vi "WILT Agilent Correct Same Voltages.vi"(11 "Standard Agilent Data":dbl[](array[numeric])=[0.0150789, 0.0067017, 0.0050262, 0.0050262, 0.0016755, 0.0067017, 0.0050262, -0.003351, -0.0050262, 0.0050262, 0.0067017, -0.0016755, 0.0134034, 0.0016755, 0.0100527, 0.0150789, 0.003351, 0.0016755, 0.0083772, 0.0150789, 0.0050262, 0.0083772, 0.0083772, 0.0100527, 0.0150789, 0.0067017, 0.0016755, 0.003351, 0.0016755, 0.0016755, 0.0134034, 0.0016755, -0.0217806, -0.0284823, 0.003351, -0.0050262, -0.0067017, 0.0134034, 0.0083772, 0.0016755, -0.0016755, 0.003351, 0.105552, 0.0234561, 0.0134034, 0.0150789, -0.0016755, -0.0016755, 0.003303, 0.0066063, -0.0016515, -0.0066063, 0.0148638, 0.0099093, -0.0016515, 0.0148638, 0.0066063, 0.003303, -0.0379854, -0.0016515, -0.0082578, -0.0049545, -0.003303, 0.0016515, -0.809256, 238.79767, 259.98711, 242.03472, 0.776226, 135.72431, 1.271691, 169.51505, 130.6045, 132.20651, 236.32036, 235.99005, 234.30546, 236.88188, -264.32902, -207.73094, 1220.801, 77.65, 348.401, 79.079, 79.717, 80.026, 78.786, 79.191, 78.937, 79.038, 80.017, 80.836, 79.409, 78.471, 79.011, 79.04, 80.102, 77.803, 77.346, 79.36, 76.685, 77.029, 77.321, 77.89, 77.27, 76.943, 78.032, 77.108, 77.549, 77.348, 79.619, 78.244, 241.03483, 243.97762, 240.40768, -3.071427, 0.0149331, 0.0099555, 0.0066369, 0.0049776, -0.0033186, 0.0, 0.0099555, 0.0082962, 0.0116148, 0.0049776, 0.0, 0.0165924, 0.0116148, 0.0033186, 0.0033186, -0.0049776, 0.0066369, 0.0066369, 0.0049776, 0.0099555, 0.0033186, 0.0165924, 0.0066369, 0.0232296, 0.0, 0.0945771, 0.0929178, 0.0016593, 0.0, 0.0099555, 0.0033186, 0.0082962, 0.0033186, 0.0099555, 0.0099555, 0.0082962, -0.0066369, -0.0116148, 0.0016593, 0.0049776, 0.0033186, 0.0066369, 0.0099555, 0.0116148, 0.0, 0.0149331, 0.0016593, 0.0066369, 77.454, 77.456, 77.632, 77.638, 77.159, 75.814, 77.922, 78.196, 78.44, 79.124, 79.366, 79.841, 80.354, 80.293, 80.037, 80.15, 79.992, 80.199, 79.751, 79.949, 80.23, 80.523, 80.593, 1072.373, 237.01965, 236.79856, 236.81435, 238.04611, 230.03965, 0.536922, 9.9e+37, 235.66154, 9.9e+37, 199.4982, 9.9e+37, 236.13531, 3.742653, 0.410586, -2.526687, -0.900132, 236.76698, 199.4982]) -> (3 "Corrected Agilent Data":dbl[](array[numeric])=[0.0150789, 0.0067017, 0.0050262, 0.0050262, 0.0016755, 0.0067017, 0.0050262, -0.003351, -0.0050262, 0.0050262, 0.0067017, -0.0016755, 0.0134034, 0.0016755, 0.0100527, 0.0150789, 0.003351, 0.0016755, 0.0083772, 0.0150789, 0.0050262, 0.0083772, 0.0083772, 0.0100527, 0.0150789, 0.0067017, 0.0016755, 0.003351, 0.0016755, 0.0016755, 0.0134034, 0.0016755, -0.0217806, -0.0284823, 0.003351, -0.0050262, -0.0067017, 0.0134034, 0.0083772, 0.0016755, -0.0016755, 0.003351, 0.105552, 0.0234561, 0.0134034, 0.0150789, -0.0016755, -0.0016755, 0.003303, 0.0066063, -0.0016515, -0.0066063, 0.0148638, 0.0099093, -0.0016515, 0.0148638, 0.0066063, 0.003303, -0.0379854, -0.0016515, -0.0082578, -0.0049545, -0.003303, 0.0016515, -0.809256, 238.79767, 259.98711, 242.03472, 0.776226, 135.72431, 1.271691, 169.51505, 130.6045, 132.20651, 236.32036, 236.32036, 236.32036, 235.99005, 235.99005, 235.99005, 234.30546, 234.30546, 234.30546, 236.88188, 236.88188, 236.88188, -264.32902, -207.73094, 1220.801, 77.65, 348.401, 79.079, 79.717, 80.026, 78.786, 79.191, 78.937, 79.038, 80.017, 80.836, 79.409, 78.471, 79.011, 79.04, 80.102, 77.803, 77.346, 79.36, 76.685, 77.029, 77.321, 77.89, 77.27, 76.943, 78.032, 77.108, 77.549, 77.348, 79.619, 78.244, 241.03483, 243.97762, 240.40768, -3.071427, 0.0149331, 0.0099555, 0.0066369, 0.0049776, -0.0033186, 0.0, 0.0099555, 0.0082962, 0.0116148, 0.0049776, 0.0, 0.0165924, 0.0116148, 0.0033186, 0.0033186, -0.0049776, 0.0066369, 0.0066369, 0.0049776, 0.0099555, 0.0033186, 0.0165924, 0.0066369, 0.0232296, 0.0, 0.0945771, 0.0929178, 0.0016593, 0.0, 0.0099555, 0.0033186, 0.0082962, 0.0033186, 0.0099555, 0.0099555, 0.0082962, -0.0066369, -0.0116148, 0.0016593, 0.0049776, 0.0033186, 0.0066369, 0.0099555, 0.0116148, 0.0, 0.0149331, 0.0016593, 0.0066369, 77.454, 77.456, 77.632, 77.638, 77.159, 75.814, 77.922, 78.196, 78.44, 79.124, 79.366, 79.841, 80.354, 80.293, 80.037, 80.15, 79.992, 80.199, 79.751, 79.949, 80.23, 80.523, 80.593, 1072.373, 237.01965, 237.01965, 237.01965, 236.79856, 236.79856, 236.79856, 236.81435, 236.81435, 236.81435, 238.04611, 238.04611, 238.04611, 230.03965, 230.03965, 230.03965, 0.536922, 9.9e+37, 235.66154, 235.66154, 235.66154, 9.9e+37, 199.4982, 9.9e+37, 236.13531, 236.13531, 236.13531, 3.742653, 0.410586, -2.526687, -0.900132, 236.76698, 236.76698, 236.76698, 199.4982])   [LabVIEW 2016]
uses:
  <vilib>/Utility/file.llb/Read From Spreadsheet File (string).vi
panel:
  out "Array":string[][](array[string])=[["LV Index", "Agilent", "Channel", "Station", "Sensor", "LV Data"], ["64", "2", "201", "5", "Volts", "-0.809256"], ["65", "2", "202", "6", "Volts", "238.797670"], ["66", "2", "203", "7", "Volts", "259.987110"], ["67", "2", "204", "8", "Volts", "242.034720"], ["68", "2", "205", "9", "Volts", "0.776226"], ["69", "2", "206", "10", "Volts", "135.724310"], ["70", "2", "207", "11", "Volts", "1.271691"], ["71", "2", "208", "12", "Volts", "169.515050"], ["72", "2", "209", "13", "Volts", "130.604500"], ["73", "2", "210", "14", "Volts", "132.206510"], ["74", "2", "211", "21", "Volts", "236.320360"], ["75", "2", "212", "24", "Volts", "235.990050"], ["76", "2", "213", "27", "Volts", "234.305460"], ["77", "2", "214", "30", "Volts", "236.881880"], ["78", "2", "215", "15", "Volts", "-264.329020"], ["79", "2", "216", "16", "Volts", "-207.730940"], ["112", "3", "313", "1", "Volts", "241.034830"], ["113", "3", "314", "2", "Volts", "243.977620"], ["114", "3", "315", "3", "Volts", "240.407680"], ["115", "3", "316", "4", "Volts", "-3.071427"], ["188", "6", "205", "33", "Volts", "237.019650"], ["189", "6", "206", "36", "Volts", "236.798560"], ["190", "6", "207", "39", "Volts", "236.814350"], ["191", "6", "208", "42", "Volts", "238.046110"], ["192", "6", "209", "45", "Volts", "230.039650"], ["193", "6", "210", "45", "Volts (208)", "0.536922"], ["195", "6", "212", "48", "Volts", "235.661540"], ["197", "6", "214", "51", "Volts (208)", "199.498200"], ["199", "6", "216", "54", "Volts", "236.135310"], ["200", "6", "301", "17", "Volts", "3.742653"], ["201", "6", "302", "18", "Volts", "0.410586"], ["202", "6", "303", "19", "Volts", "-2.526687"], ["203", "6", "304", "20", "Volts", "-0.900132"], ["204", "6", "305", "51", "Volts", "236.766980"], ["205", "6", "306", "48", "Volts (208)", "199.498200"]]
  in  "Initial Output Array 2":string[][](array[string])=[["LV Index", "Agilent", "Channel", "Station", "Sensor", "LV Data"], ["0", "1", "101", "1", "L1 Current", "0.015079"], ["1", "1", "102", "1", "L2 Current", "0.006702"], ["2", "1", "103", "2", "L1 Current", "0.005026"], ["3", "1", "104", "2", "L2 Current", "0.005026"], ["4", "1", "105", "3", "L1 Current", "0.001675"], ["5", "1", "106", "3", "L2 Current", "0.006702"], ["6", "1", "107", "4", "L1 Current", "0.005026"], ["7", "1", "108", "4", "L2 Current", "-0.003351"], ["8", "1", "109", "5", "L1 Current", "-0.005026"], ["9", "1", "110", "5", "L2 Current", "0.005026"], ["10", "1", "111", "6", "L1 Current", "0.006702"], ["11", "1", "112", "6", "L2 Current", "-0.001675"], ["12", "1", "113", "7", "L1 Current", "0.013403"], ["13", "1", "114", "7", "L2 Current", "0.001675"], ["14", "1", "115", "8", "L1 Current", "0.010053"], ["15", "1", "116", "8", "L2 Current", "0.015079"], ["16", "1", "201", "9", "L1 Current", "0.003351"], ["17", "1", "202", "9", "L2 Current", "0.001675"], ["18", "1", "203", "10", "L1 Current", "0.008377"], ["19", "1", "204", "10", "L2 Current", "0.015079"], ["20", "1", "205", "11", "L1 Current", "0.005026"], ["21", "1", "206", "11", "L2 Current", "0.008377"], ["22", "1", "207", "12", "L1 Current", "0.008377"], ["23", "1", "208", "12", "L2 Current", "0.010053"], ["24", "1", "209", "13", "L1 Current", "0.015079"], ["25", "1", "210", "13", "L2 Current", "0.006702"], ["26", "1", "211", "14", "L1 Current", "0.001675"], ["27", "1", "212", "14", "L2 Current", "0.003351"], ["28", "1", "213", "15", "L1 Current", "0.001675"], ["29", "1", "214", "15", "L2 Current", "0.001675"], ["30", "1", "215", "16", "L1 Current", "0.013403"], ["31", "1", "216", "16", "L2 Current", "0.001675"], ["32", "1", "301", "17", "L1 Current", "-0.021781"], ["33", "1", "302", "17", "L2 Current", "-0.028482"], ["34", "1", "303", "18", "L1 Current", "0.003351"], ["35", "1", "304", "18", "L2 Current", "-0.005026"], ["36", "1", "305", "19", "L1 Current", "-0.006702"], ["37", "1", "306", "19", "L2 Current", "0.013403"], ["38", "1", "307", "20", "L1 Current", "0.008377"], ["39", "1", "308", "20", "L2 Current", "0.001675"], ["40", "1", "309", "21", "L1 Current", "-0.001675"], ["41", "1", "310", "21", "L2 Current", "0.003351"], ["42", "1", "311", "22", "L1 Current", "0.105552"], ["43", "1", "312", "22", "L2 Current", "0.023456"], ["44", "1", "313", "23", "L1 Current", "0.013403"], ["45", "1", "314", "23", "L2 Current", "0.015079"], ["46", "1", "315", "24", "L1 Current", "-0.001675"], ["47", "1", "316", "24", "L2 Current", "-0.001675"], ["48", "2", "101", "25", "L1 Current", "0.003303"], ["49", "2", "102", "25", "L2 Current", "0.006606"], ["50", "2", "103", "26", "L1 Current", "-0.001651"], ["51", "2", "104", "26", "L2 Current", "-0.006606"], ["52", "2", "105", "27", "L1 Current", "0.014864"], ["53", "2", "106", "27", "L2 Current", "0.009909"], ["54", "2", "107", "28", "L1 Current", "-0.001651"], ["55", "2", "108", "28", "L2 Current", "0.014864"], ["56", "2", "109", "29", "L1 Current", "0.006606"], ["57", "2", "110", "29", "L2 Current", "0.003303"], ["58", "2", "111", "30", "L1 Current", "-0.037985"], ["59", "2", "112", "30", "L2 Current", "-0.001651"], ["60", "2", "113", "31", "L1 Current", "-0.008258"], ["61", "2", "114", "31", "L2 Current", "-0.004954"], ["62", "2", "115", "32", "L1 Current", "-0.003303"], ["63", "2", "116", "32", "L2 Current", "0.001651"], ["64", "2", "201", "5", "Volts", "-0.809256"], ["65", "2", "202", "6", "Volts", "238.797670"], ["66", "2", "203", "7", "Volts", "259.987110"], ["67", "2", "204", "8", "Volts", "242.034720"], ["68", "2", "205", "9", "Volts", "0.776226"], ["69", "2", "206", "10", "Volts", "135.724310"], ["70", "2", "207", "11", "Volts", "1.271691"], ["71", "2", "208", "12", "Volts", "169.515050"], ["72", "2", "209", "13", "Volts", "130.604500"], ["73", "2", "210", "14", "Volts", "132.206510"], ["74", "2", "211", "21", "Volts", "236.320360"], ["75", "2", "212", "24", "Volts", "235.990050"], ["76", "2", "213", "27", "Volts", "234.305460"], ["77", "2", "214", "30", "Volts", "236.881880"], ["78", "2", "215", "15", "Volts", "-264.329020"], ["79", "2", "216", "16", "Volts", "-207.730940"], ["80", "3", "201", "1", "Temperature", "1220.801000"], ["81", "3", "202", "2", "Temperature", "77.650000"], ["82", "3", "203", "3", "Temperature", "348.401000"], ["83", "3", "204", "4", "Temperature", "79.079000"], ["84", "3", "205", "5", "Temperature", "79.717000"], ["85", "3", "206", "6", "Temperature", "80.026000"], ["86", "3", "207", "7", "Temperature", "78.786000"], ["87", "3", "208", "8", "Temperature", "79.191000"], ["88", "3", "209", "9", "Temperature", "78.937000"], ["89", "3", "210", "10", "Temperature", "79.038000"], ["90", "3", "211", "11", "Temperature", "80.017000"], ["91", "3", "212", "12", "Temperature", "80.836000"], ["92", "3", "213", "13", "Temperature", "79.409000"], ["93", "3", "214", "14", "Temperature", "78.471000"], ["94", "3", "215", "15", "Temperature", "79.011000"], ["95", "3", "216", "16", "Temperature", "79.040000"], ["96", "3", "217", "17", "Temperature", "80.102000"], ["97", "3", "218", "18", "Temperature", "77.803000"], ["98", "3", "219", "19", "Temperature", "77.346000"], ["99", "3", "220", "20", "Temperature", "79.360000"], ["100", "3", "301", "21", "Temperature", "76.685000"], ["101", "3", "302", "22", "Temperature", "77.029000"], ["102", "3", "303", "23", "Temperature", "77.321000"], ["103", "3", "304", "24", "Temperature", "77.890000"], ["104", "3", "305", "25", "Temperature", "77.270000"], ["105", "3", "306", "26", "Temperature", "76.943000"], ["106", "3", "307", "27", "Temperature", "78.032000"], ["107", "3", "308", "28", "Temperature", "77.108000"], ["108", "3", "309", "29", "Temperature", "77.549000"], ["109", "3", "310", "30", "Temperature", "77.348000"], ["110", "3", "311", "31", "Temperature", "79.619000"], ["111", "3", "312", "32", "Temperature", "78.244000"], ["112", "3", "313", "1", "Volts", "241.034830"], ["113", "3", "314", "2", "Volts", "243.977620"], ["114", "3", "315", "3", "Volts", "240.407680"], ["115", "3", "316", "4", "Volts", "-3.071427"], ["116", "4", "101", "33", "L1 Current", "0.014933"], ["117", "4", "102", "33", "L2 Current", "0.009956"], ["118", "4", "103", "34", "L1 Current", "0.006637"], ["119", "4", "104", "34", "L2 Current", "0.004978"], ["120", "4", "105", "35", "L1 Current", "-0.003319"], ["121", "4", "106", "35", "L2 Current", "0.000000"], ["122", "4", "107", "36", "L1 Current", "0.009956"], ["123", "4", "108", "36", "L2 Current", "0.008296"], ["124", "4", "109", "37", "L1 Current", "0.011615"], ["125", "4", "110", "37", "L2 Current", "0.004978"], ["126", "4", "111", "38", "L1 Current", "0.000000"], ["127", "4", "112", "38", "L2 Current", "0.016592"], ["128", "4", "113", "39", "L1 Current", "0.011615"], ["129", "4", "114", "39", "L2 Current", "0.003319"], ["130", "4", "115", "40", "L1 Current", "0.003319"], ["131", "4", "116", "40", "L2 Current", "-0.004978"], ["132", "4", "201", "41", "L1 Current", "0.006637"], ["133", "4", "202", "41", "L2 Current", "0.006637"], ["134", "4", "203", "42", "L1 Current", "0.004978"], ["135", "4", "204", "42", "L2 Current", "0.009956"], ["136", "4", "205", "43", "L1 Current", "0.003319"], ["137", "4", "206", "43", "L2 Current", "0.016592"], ["138", "4", "207", "44", "L1 Current", "0.006637"], ["139", "4", "208", "44", "L2 Current", "0.023230"], ["140", "4", "209", "45", "L1 Current", "0.000000"], ["141", "4", "210", "45", "L2 Current", "0.094577"], ["142", "4", "211", "46", "L1 Current", "0.092918"], ["143", "4", "212", "46", "L2 Current", "0.001659"], ["144", "4", "213", "47", "L1 Current", "0.000000"], ["145", "4", "214", "47", "L2 Current", "0.009956"], ["146", "4", "215", "48", "L1 Current", "0.003319"], ["147", "4", "216", "48", "L2 Current", "0.008296"], ["148", "4", "301", "49", "L1 Current", "0.003319"], ["149", "4", "302", "49", "L2 Current", "0.009956"], ["150", "4", "303", "50", "L1 Current", "0.009956"], ["151", "4", "304", "50", "L2 Current", "0.008296"], ["152", "4", "305", "51", "L1 Current", "-0.006637"], ["153", "4", "306", "51", "L2 Current", "-0.011615"], ["154", "4", "307", "52", "L1 Current", "0.001659"], ["155", "4", "308", "52", "L2 Current", "0.004978"], ["156", "4", "309", "53", "L1 Current", "0.003319"], ["157", "4", "310", "53", "L2 Current", "0.006637"], ["158", "4", "311", "54", "L1 Current", "0.009956"], ["159", "4", "312", "54", "L2 Current", "0.011615"], ["160", "4", "313", "55", "L1 Current", "0.000000"], ["161", "4", "314", "55", "L2 Current", "0.014933"], ["162", "4", "315", "56", "L1 Current", "0.001659"], ["163", "4", "316", "56", "L2 Current", "0.006637"], ["164", "6", "101", "33", "Temperature", "77.454000"], ["165", "6", "102", "34", "Temperature", "77.456000"], ["166", "6", "103", "35", "Temperature", "77.632000"], ["167", "6", "104", "36", "Temperature", "77.638000"], ["168", "6", "105", "37", "Temperature", "77.159000"], ["169", "6", "106", "38", "Temperature", "75.814000"], ["170", "6", "107", "39", "Temperature", "77.922000"], ["171", "6", "108", "40", "Temperature", "78.196000"], ["172", "6", "109", "41", "Temperature", "78.440000"], ["173", "6", "110", "42", "Temperature", "79.124000"], ["174", "6", "111", "43", "Temperature", "79.366000"], ["175", "6", "112", "44", "Temperature", "79.841000"], ["176", "6", "113", "45", "Temperature", "80.354000"], ["177", "6", "114", "46", "Temperature", "80.293000"], ["178", "6", "115", "47", "Temperature", "80.037000"], ["179", "6", "116", "48", "Temperature", "80.150000"], ["180", "6", "117", "49", "Temperature", "79.992000"], ["181", "6", "118", "50", "Temperature", "80.199000"], ["182", "6", "119", "51", "Temperature", "79.751000"], ["183", "6", "120", "52", "Temperature", "79.949000"], ["184", "6", "201", "53", "Temperature", "80.230000"], ["185", "6", "202", "54", "Temperature", "80.523000"], ["186", "6", "203", "55", "Temperature", "80.593000"], ["187", "6", "204", "56", "Temperature", "1072.373000"], ["188", "6", "205", "33", "Volts", "237.019650"], ["189", "6", "206", "36", "Volts", "236.798560"], ["190", "6", "207", "39", "Volts", "236.814350"], ["191", "6", "208", "42", "Volts", "238.046110"], ["192", "6", "209", "45", "Volts", "230.039650"], ["193", "6", "210", "45", "Volts (208)", "0.536922"], ["194", "6", "211", "45", "SW (208)", "98999999999999993400000000000000000000.000000"], ["195", "6", "212", "48", "Volts", "235.661540"], ["196", "6", "213", "48", "SW (208)", "98999999999999993400000000000000000000.000000"], ["197", "6", "214", "51", "Volts (208)", "199.498200"], ["198", "6", "215", "51", "SW (208)", "98999999999999993400000000000000000000.000000"], ["199", "6", "216", "54", "Volts", "236.135310"], ["200", "6", "301", "17", "Volts", "3.742653"], ["201", "6", "302", "18", "Volts", "0.410586"], ["202", "6", "303", "19", "Volts", "-2.526687"], ["203", "6", "304", "20", "Volts", "-0.900132"], ["204", "6", "305", "51", "Volts", "236.766980"], ["205", "6", "306", "48", "Volts (208)", "199.498200"]]
  out "Final output array":string[][](array[string])=[["LabView Array Index", "Agilent", "Channel", "Station", "Sensor", "LV Data"], ["0", "1", "101", "1", "L1 Current", "0.015079"], ["1", "1", "102", "1", "L2 Current", "0.006702"], ["2", "1", "103", "2", "L1 Current", "0.005026"], ["3", "1", "104", "2", "L2 Current", "0.005026"], ["4", "1", "105", "3", "L1 Current", "0.001675"], ["5", "1", "106", "3", "L2 Current", "0.006702"], ["6", "1", "107", "4", "L1 Current", "0.005026"], ["7", "1", "108", "4", "L2 Current", "-0.003351"], ["8", "1", "109", "5", "L1 Current", "-0.005026"], ["9", "1", "110", "5", "L2 Current", "0.005026"], ["10", "1", "111", "6", "L1 Current", "0.006702"], ["11", "1", "112", "6", "L2 Current", "-0.001675"], ["12", "1", "113", "7", "L1 Current", "0.013403"], ["13", "1", "114", "7", "L2 Current", "0.001675"], ["14", "1", "115", "8", "L1 Current", "0.010053"], ["15", "1", "116", "8", "L2 Current", "0.015079"], ["16", "1", "201", "9", "L1 Current", "0.003351"], ["17", "1", "202", "9", "L2 Current", "0.001675"], ["18", "1", "203", "10", "L1 Current", "0.008377"], ["19", "1", "204", "10", "L2 Current", "0.015079"], ["20", "1", "205", "11", "L1 Current", "0.005026"], ["21", "1", "206", "11", "L2 Current", "0.008377"], ["22", "1", "207", "12", "L1 Current", "0.008377"], ["23", "1", "208", "12", "L2 Current", "0.010053"], ["24", "1", "209", "13", "L1 Current", "0.015079"], ["25", "1", "210", "13", "L2 Current", "0.006702"], ["26", "1", "211", "14", "L1 Current", "0.001675"], ["27", "1", "212", "14", "L2 Current", "0.003351"], ["28", "1", "213", "15", "L1 Current", "0.001675"], ["29", "1", "214", "15", "L2 Current", "0.001675"], ["30", "1", "215", "16", "L1 Current", "0.013403"], ["31", "1", "216", "16", "L2 Current", "0.001675"], ["32", "1", "301", "17", "L1 Current", "-0.021781"], ["33", "1", "302", "17", "L2 Current", "-0.028482"], ["34", "1", "303", "18", "L1 Current", "0.003351"], ["35", "1", "304", "18", "L2 Current", "-0.005026"], ["36", "1", "305", "19", "L1 Current", "-0.006702"], ["37", "1", "306", "19", "L2 Current", "0.013403"], ["38", "1", "307", "20", "L1 Current", "0.008377"], ["39", "1", "308", "20", "L2 Current", "0.001675"], ["40", "1", "309", "21", "L1 Current", "-0.001675"], ["41", "1", "310", "21", "L2 Current", "0.003351"], ["42", "1", "311", "22", "L1 Current", "0.105552"], ["43", "1", "312", "22", "L2 Current", "0.023456"], ["44", "1", "313", "23", "L1 Current", "0.013403"], ["45", "1", "314", "23", "L2 Current", "0.015079"], ["46", "1", "315", "24", "L1 Current", "-0.001675"], ["47", "1", "316", "24", "L2 Current", "-0.001675"], ["48", "2", "101", "25", "L1 Current", "0.003303"], ["49", "2", "102", "25", "L2 Current", "0.006606"], ["50", "2", "103", "26", "L1 Current", "-0.001651"], ["51", "2", "104", "26", "L2 Current", "-0.006606"], ["52", "2", "105", "27", "L1 Current", "0.014864"], ["53", "2", "106", "27", "L2 Current", "0.009909"], ["54", "2", "107", "28", "L1 Current", "-0.001651"], ["55", "2", "108", "28", "L2 Current", "0.014864"], ["56", "2", "109", "29", "L1 Current", "0.006606"], ["57", "2", "110", "29", "L2 Current", "0.003303"], ["58", "2", "111", "30", "L1 Current", "-0.037985"], ["59", "2", "112", "30", "L2 Current", "-0.001651"], ["60", "2", "113", "31", "L1 Current", "-0.008258"], ["61", "2", "114", "31", "L2 Current", "-0.004954"], ["62", "2", "115", "32", "L1 Current", "-0.003303"], ["63", "2", "116", "32", "L2 Current", "0.001651"], ["64", "2", "201", "5", "Volts", "-0.809256"], ["65", "2", "202", "6", "Volts", "238.797670"], ["66", "2", "203", "7", "Volts", "259.987110"], ["67", "2", "204", "8", "Volts", "242.034720"], ["68", "2", "205", "9", "Volts", "0.776226"], ["69", "2", "206", "10", "Volts", "135.724310"], ["70", "2", "207", "11", "Volts", "1.271691"], ["71", "2", "208", "12", "Volts", "169.515050"], ["72", "2", "209", "13", "Volts", "130.604500"], ["73", "2", "210", "14", "Volts", "132.206510"], ["74", "2", "211", "21", "Volts", "236.320360"], ["74", "2", "211", "22", "Volts", "236.320360"], ["74", "2", "211", "23", "Volts", "236.320360"], ["75", "2", "212", "24", "Volts", "235.990050"], ["75", "2", "212", "25", "Volts", "235.990050"], ["75", "2", "212", "26", "Volts", "235.990050"], ["76", "2", "213", "27", "Volts", "234.305460"], ["76", "2", "213", "28", "Volts", "234.305460"], ["76", "2", "213", "29", "Volts", "234.305460"], ["77", "2", "214", "30", "Volts", "236.881880"], ["77", "2", "214", "31", "Volts", "236.881880"], ["77", "2", "214", "32", "Volts", "236.881880"], ["78", "2", "215", "15", "Volts", "-264.329020"], ["79", "2", "216", "16", "Volts", "-207.730940"], ["80", "3", "201", "1", "Temperature", "1220.801000"], ["81", "3", "202", "2", "Temperature", "77.650000"], ["82", "3", "203", "3", "Temperature", "348.401000"], ["83", "3", "204", "4", "Temperature", "79.079000"], ["84", "3", "205", "5", "Temperature", "79.717000"], ["85", "3", "206", "6", "Temperature", "80.026000"], ["86", "3", "207", "7", "Temperature", "78.786000"], ["87", "3", "208", "8", "Temperature", "79.191000"], ["88", "3", "209", "9", "Temperature", "78.937000"], ["89", "3", "210", "10", "Temperature", "79.038000"], ["90", "3", "211", "11", "Temperature", "80.017000"], ["91", "3", "212", "12", "Temperature", "80.836000"], ["92", "3", "213", "13", "Temperature", "79.409000"], ["93", "3", "214", "14", "Temperature", "78.471000"], ["94", "3", "215", "15", "Temperature", "79.011000"], ["95", "3", "216", "16", "Temperature", "79.040000"], ["96", "3", "217", "17", "Temperature", "80.102000"], ["97", "3", "218", "18", "Temperature", "77.803000"], ["98", "3", "219", "19", "Temperature", "77.346000"], ["99", "3", "220", "20", "Temperature", "79.360000"], ["100", "3", "301", "21", "Temperature", "76.685000"], ["101", "3", "302", "22", "Temperature", "77.029000"], ["102", "3", "303", "23", "Temperature", "77.321000"], ["103", "3", "304", "24", "Temperature", "77.890000"], ["104", "3", "305", "25", "Temperature", "77.270000"], ["105", "3", "306", "26", "Temperature", "76.943000"], ["106", "3", "307", "27", "Temperature", "78.032000"], ["107", "3", "308", "28", "Temperature", "77.108000"], ["108", "3", "309", "29", "Temperature", "77.549000"], ["109", "3", "310", "30", "Temperature", "77.348000"], ["110", "3", "311", "31", "Temperature", "79.619000"], ["111", "3", "312", "32", "Temperature", "78.244000"], ["112", "3", "313", "1", "Volts", "241.034830"], ["113", "3", "314", "2", "Volts", "243.977620"], ["114", "3", "315", "3", "Volts", "240.407680"], ["115", "3", "316", "4", "Volts", "-3.071427"], ["116", "4", "101", "33", "L1 Current", "0.014933"], ["117", "4", "102", "33", "L2 Current", "0.009956"], ["118", "4", "103", "34", "L1 Current", "0.006637"], ["119", "4", "104", "34", "L2 Current", "0.004978"], ["120", "4", "105", "35", "L1 Current", "-0.003319"], ["121", "4", "106", "35", "L2 Current", "0.000000"], ["122", "4", "107", "36", "L1 Current", "0.009956"], ["123", "4", "108", "36", "L2 Current", "0.008296"], ["124", "4", "109", "37", "L1 Current", "0.011615"], ["125", "4", "110", "37", "L2 Current", "0.004978"], ["126", "4", "111", "38", "L1 Current", "0.000000"], ["127", "4", "112", "38", "L2 Current", "0.016592"], ["128", "4", "113", "39", "L1 Current", "0.011615"], ["129", "4", "114", "39", "L2 Current", "0.003319"], ["130", "4", "115", "40", "L1 Current", "0.003319"], ["131", "4", "116", "40", "L2 Current", "-0.004978"], ["132", "4", "201", "41", "L1 Current", "0.006637"], ["133", "4", "202", "41", "L2 Current", "0.006637"], ["134", "4", "203", "42", "L1 Current", "0.004978"], ["135", "4", "204", "42", "L2 Current", "0.009956"], ["136", "4", "205", "43", "L1 Current", "0.003319"], ["137", "4", "206", "43", "L2 Current", "0.016592"], ["138", "4", "207", "44", "L1 Current", "0.006637"], ["139", "4", "208", "44", "L2 Current", "0.023230"], ["140", "4", "209", "45", "L1 Current", "0.000000"], ["141", "4", "210", "45", "L2 Current", "0.094577"], ["142", "4", "211", "46", "L1 Current", "0.092918"], ["143", "4", "212", "46", "L2 Current", "0.001659"], ["144", "4", "213", "47", "L1 Current", "0.000000"], ["145", "4", "214", "47", "L2 Current", "0.009956"], ["146", "4", "215", "48", "L1 Current", "0.003319"], ["147", "4", "216", "48", "L2 Current", "0.008296"], ["148", "4", "301", "49", "L1 Current", "0.003319"], ["149", "4", "302", "49", "L2 Current", "0.009956"], ["150", "4", "303", "50", "L1 Current", "0.009956"], ["151", "4", "304", "50", "L2 Current", "0.008296"], ["152", "4", "305", "51", "L1 Current", "-0.006637"], ["153", "4", "306", "51", "L2 Current", "-0.011615"], ["154", "4", "307", "52", "L1 Current", "0.001659"], ["155", "4", "308", "52", "L2 Current", "0.004978"], ["156", "4", "309", "53", "L1 Current", "0.003319"], ["157", "4", "310", "53", "L2 Current", "0.006637"], ["158", "4", "311", "54", "L1 Current", "0.009956"], ["159", "4", "312", "54", "L2 Current", "0.011615"], ["160", "4", "313", "55", "L1 Current", "0.000000"], ["161", "4", "314", "55", "L2 Current", "0.014933"], ["162", "4", "315", "56", "L1 Current", "0.001659"], ["163", "4", "316", "56", "L2 Current", "0.006637"], ["164", "6", "101", "33", "Temperature", "77.454000"], ["165", "6", "102", "34", "Temperature", "77.456000"], ["166", "6", "103", "35", "Temperature", "77.632000"], ["167", "6", "104", "36", "Temperature", "77.638000"], ["168", "6", "105", "37", "Temperature", "77.159000"], ["169", "6", "106", "38", "Temperature", "75.814000"], ["170", "6", "107", "39", "Temperature", "77.922000"], ["171", "6", "108", "40", "Temperature", "78.196000"], ["172", "6", "109", "41", "Temperature", "78.440000"], ["173", "6", "110", "42", "Temperature", "79.124000"], ["174", "6", "111", "43", "Temperature", "79.366000"], ["175", "6", "112", "44", "Temperature", "79.841000"], ["176", "6", "113", "45", "Temperature", "80.354000"], ["177", "6", "114", "46", "Temperature", "80.293000"], ["178", "6", "115", "47", "Temperature", "80.037000"], ["179", "6", "116", "48", "Temperature", "80.150000"], ["180", "6", "117", "49", "Temperature", "79.992000"], ["181", "6", "118", "50", "Temperature", "80.199000"], ["182", "6", "119", "51", "Temperature", "79.751000"], ["183", "6", "120", "52", "Temperature", "79.949000"], ["184", "6", "201", "53", "Temperature", "80.230000"], ["185", "6", "202", "54", "Temperature", "80.523000"], ["186", "6", "203", "55", "Temperature", "80.593000"], ["187", "6", "204", "56", "Temperature", "1072.373000"], ["188", "6", "205", "33", "Volts", "237.019650"], ["188", "6", "205", "34", "Volts", "237.019650"], ["188", "6", "205", "35", "Volts", "237.019650"], ["189", "6", "206", "36", "Volts", "236.798560"], ["189", "6", "206", "37", "Volts", "236.798560"], ["189", "6", "206", "38", "Volts", "236.798560"], ["190", "6", "207", "39", "Volts", "236.814350"], ["190", "6", "207", "40", "Volts", "236.814350"], ["191", "6", "208", "42", "Volts", "236.814350"], ["191", "6", "208", "43", "Volts", "238.046110"], ["191", "6", "208", "44", "Volts", "238.046110"], ["192", "6", "209", "45", "Volts", "238.046110"], ["192", "6", "209", "46", "Volts", "230.039650"], ["192", "6", "209", "47", "Volts", "230.039650"], ["193", "6", "210", "45", "Volts (208)", "230.039650"], ["194", "6", "211", "45", "SW (208)", "0.536922"], ["195", "6", "212", "48", "Volts", "98999999999999993400000000000000000000.000000"], ["195", "6", "212", "49", "Volts", "235.661540"], ["195", "6", "212", "50", "Volts", "235.661540"], ["196", "6", "213", "48", "SW (208)", "235.661540"], ["197", "6", "214", "51", "Volts (208)", "98999999999999993400000000000000000000.000000"], ["198", "6", "215", "51", "SW (208)", "199.498200"], ["199", "6", "216", "54", "Volts", "98999999999999993400000000000000000000.000000"], ["199", "6", "216", "55", "Volts", "236.135310"], ["199", "6", "216", "56", "Volts", "236.135310"], ["200", "6", "301", "17", "Volts", "236.135310"], ["201", "6", "302", "18", "Volts", "3.742653"], ["202", "6", "303", "19", "Volts", "0.410586"], ["203", "6", "304", "20", "Volts", "-2.526687"], ["204", "6", "305", "51", "Volts", "-0.900132"], ["204", "6", "305", "52", "Volts", "236.766980"], ["204", "6", "305", "53", "Volts", "236.766980"], ["205", "6", "306", "48", "Volts (208)", "236.766980"]]
  in  "file path (dialog if empty) 2":path=path "C:/Users/220038920/Desktop/Project/NI-2010/Trunk/Dryer Wilt/Documentation/Agilent Array Names DUP.csv"
  out "Initial Output Array":string[][](array[string])=[["LV Index", "Agilent", "Channel", "Station", "Sensor", "LV Data"], ["0", "1", "101", "1", "L1 Current", "0.015079"], ["1", "1", "102", "1", "L2 Current", "0.006702"], ["2", "1", "103", "2", "L1 Current", "0.005026"], ["3", "1", "104", "2", "L2 Current", "0.005026"], ["4", "1", "105", "3", "L1 Current", "0.001675"], ["5", "1", "106", "3", "L2 Current", "0.006702"], ["6", "1", "107", "4", "L1 Current", "0.005026"], ["7", "1", "108", "4", "L2 Current", "-0.003351"], ["8", "1", "109", "5", "L1 Current", "-0.005026"], ["9", "1", "110", "5", "L2 Current", "0.005026"], ["10", "1", "111", "6", "L1 Current", "0.006702"], ["11", "1", "112", "6", "L2 Current", "-0.001675"], ["12", "1", "113", "7", "L1 Current", "0.013403"], ["13", "1", "114", "7", "L2 Current", "0.001675"], ["14", "1", "115", "8", "L1 Current", "0.010053"], ["15", "1", "116", "8", "L2 Current", "0.015079"], ["16", "1", "201", "9", "L1 Current", "0.003351"], ["17", "1", "202", "9", "L2 Current", "0.001675"], ["18", "1", "203", "10", "L1 Current", "0.008377"], ["19", "1", "204", "10", "L2 Current", "0.015079"], ["20", "1", "205", "11", "L1 Current", "0.005026"], ["21", "1", "206", "11", "L2 Current", "0.008377"], ["22", "1", "207", "12", "L1 Current", "0.008377"], ["23", "1", "208", "12", "L2 Current", "0.010053"], ["24", "1", "209", "13", "L1 Current", "0.015079"], ["25", "1", "210", "13", "L2 Current", "0.006702"], ["26", "1", "211", "14", "L1 Current", "0.001675"], ["27", "1", "212", "14", "L2 Current", "0.003351"], ["28", "1", "213", "15", "L1 Current", "0.001675"], ["29", "1", "214", "15", "L2 Current", "0.001675"], ["30", "1", "215", "16", "L1 Current", "0.013403"], ["31", "1", "216", "16", "L2 Current", "0.001675"], ["32", "1", "301", "17", "L1 Current", "-0.021781"], ["33", "1", "302", "17", "L2 Current", "-0.028482"], ["34", "1", "303", "18", "L1 Current", "0.003351"], ["35", "1", "304", "18", "L2 Current", "-0.005026"], ["36", "1", "305", "19", "L1 Current", "-0.006702"], ["37", "1", "306", "19", "L2 Current", "0.013403"], ["38", "1", "307", "20", "L1 Current", "0.008377"], ["39", "1", "308", "20", "L2 Current", "0.001675"], ["40", "1", "309", "21", "L1 Current", "-0.001675"], ["41", "1", "310", "21", "L2 Current", "0.003351"], ["42", "1", "311", "22", "L1 Current", "0.105552"], ["43", "1", "312", "22", "L2 Current", "0.023456"], ["44", "1", "313", "23", "L1 Current", "0.013403"], ["45", "1", "314", "23", "L2 Current", "0.015079"], ["46", "1", "315", "24", "L1 Current", "-0.001675"], ["47", "1", "316", "24", "L2 Current", "-0.001675"], ["48", "2", "101", "25", "L1 Current", "0.003303"], ["49", "2", "102", "25", "L2 Current", "0.006606"], ["50", "2", "103", "26", "L1 Current", "-0.001651"], ["51", "2", "104", "26", "L2 Current", "-0.006606"], ["52", "2", "105", "27", "L1 Current", "0.014864"], ["53", "2", "106", "27", "L2 Current", "0.009909"], ["54", "2", "107", "28", "L1 Current", "-0.001651"], ["55", "2", "108", "28", "L2 Current", "0.014864"], ["56", "2", "109", "29", "L1 Current", "0.006606"], ["57", "2", "110", "29", "L2 Current", "0.003303"], ["58", "2", "111", "30", "L1 Current", "-0.037985"], ["59", "2", "112", "30", "L2 Current", "-0.001651"], ["60", "2", "113", "31", "L1 Current", "-0.008258"], ["61", "2", "114", "31", "L2 Current", "-0.004954"], ["62", "2", "115", "32", "L1 Current", "-0.003303"], ["63", "2", "116", "32", "L2 Current", "0.001651"], ["64", "2", "201", "5", "Volts", "-0.809256"], ["65", "2", "202", "6", "Volts", "238.797670"], ["66", "2", "203", "7", "Volts", "259.987110"], ["67", "2", "204", "8", "Volts", "242.034720"], ["68", "2", "205", "9", "Volts", "0.776226"], ["69", "2", "206", "10", "Volts", "135.724310"], ["70", "2", "207", "11", "Volts", "1.271691"], ["71", "2", "208", "12", "Volts", "169.515050"], ["72", "2", "209", "13", "Volts", "130.604500"], ["73", "2", "210", "14", "Volts", "132.206510"], ["74", "2", "211", "21", "Volts", "236.320360"], ["75", "2", "212", "24", "Volts", "235.990050"], ["76", "2", "213", "27", "Volts", "234.305460"], ["77", "2", "214", "30", "Volts", "236.881880"], ["78", "2", "215", "15", "Volts", "-264.329020"], ["79", "2", "216", "16", "Volts", "-207.730940"], ["80", "3", "201", "1", "Temperature", "1220.801000"], ["81", "3", "202", "2", "Temperature", "77.650000"], ["82", "3", "203", "3", "Temperature", "348.401000"], ["83", "3", "204", "4", "Temperature", "79.079000"], ["84", "3", "205", "5", "Temperature", "79.717000"], ["85", "3", "206", "6", "Temperature", "80.026000"], ["86", "3", "207", "7", "Temperature", "78.786000"], ["87", "3", "208", "8", "Temperature", "79.191000"], ["88", "3", "209", "9", "Temperature", "78.937000"], ["89", "3", "210", "10", "Temperature", "79.038000"], ["90", "3", "211", "11", "Temperature", "80.017000"], ["91", "3", "212", "12", "Temperature", "80.836000"], ["92", "3", "213", "13", "Temperature", "79.409000"], ["93", "3", "214", "14", "Temperature", "78.471000"], ["94", "3", "215", "15", "Temperature", "79.011000"], ["95", "3", "216", "16", "Temperature", "79.040000"], ["96", "3", "217", "17", "Temperature", "80.102000"], ["97", "3", "218", "18", "Temperature", "77.803000"], ["98", "3", "219", "19", "Temperature", "77.346000"], ["99", "3", "220", "20", "Temperature", "79.360000"], ["100", "3", "301", "21", "Temperature", "76.685000"], ["101", "3", "302", "22", "Temperature", "77.029000"], ["102", "3", "303", "23", "Temperature", "77.321000"], ["103", "3", "304", "24", "Temperature", "77.890000"], ["104", "3", "305", "25", "Temperature", "77.270000"], ["105", "3", "306", "26", "Temperature", "76.943000"], ["106", "3", "307", "27", "Temperature", "78.032000"], ["107", "3", "308", "28", "Temperature", "77.108000"], ["108", "3", "309", "29", "Temperature", "77.549000"], ["109", "3", "310", "30", "Temperature", "77.348000"], ["110", "3", "311", "31", "Temperature", "79.619000"], ["111", "3", "312", "32", "Temperature", "78.244000"], ["112", "3", "313", "1", "Volts", "241.034830"], ["113", "3", "314", "2", "Volts", "243.977620"], ["114", "3", "315", "3", "Volts", "240.407680"], ["115", "3", "316", "4", "Volts", "-3.071427"], ["116", "4", "101", "33", "L1 Current", "0.014933"], ["117", "4", "102", "33", "L2 Current", "0.009956"], ["118", "4", "103", "34", "L1 Current", "0.006637"], ["119", "4", "104", "34", "L2 Current", "0.004978"], ["120", "4", "105", "35", "L1 Current", "-0.003319"], ["121", "4", "106", "35", "L2 Current", "0.000000"], ["122", "4", "107", "36", "L1 Current", "0.009956"], ["123", "4", "108", "36", "L2 Current", "0.008296"], ["124", "4", "109", "37", "L1 Current", "0.011615"], ["125", "4", "110", "37", "L2 Current", "0.004978"], ["126", "4", "111", "38", "L1 Current", "0.000000"], ["127", "4", "112", "38", "L2 Current", "0.016592"], ["128", "4", "113", "39", "L1 Current", "0.011615"], ["129", "4", "114", "39", "L2 Current", "0.003319"], ["130", "4", "115", "40", "L1 Current", "0.003319"], ["131", "4", "116", "40", "L2 Current", "-0.004978"], ["132", "4", "201", "41", "L1 Current", "0.006637"], ["133", "4", "202", "41", "L2 Current", "0.006637"], ["134", "4", "203", "42", "L1 Current", "0.004978"], ["135", "4", "204", "42", "L2 Current", "0.009956"], ["136", "4", "205", "43", "L1 Current", "0.003319"], ["137", "4", "206", "43", "L2 Current", "0.016592"], ["138", "4", "207", "44", "L1 Current", "0.006637"], ["139", "4", "208", "44", "L2 Current", "0.023230"], ["140", "4", "209", "45", "L1 Current", "0.000000"], ["141", "4", "210", "45", "L2 Current", "0.094577"], ["142", "4", "211", "46", "L1 Current", "0.092918"], ["143", "4", "212", "46", "L2 Current", "0.001659"], ["144", "4", "213", "47", "L1 Current", "0.000000"], ["145", "4", "214", "47", "L2 Current", "0.009956"], ["146", "4", "215", "48", "L1 Current", "0.003319"], ["147", "4", "216", "48", "L2 Current", "0.008296"], ["148", "4", "301", "49", "L1 Current", "0.003319"], ["149", "4", "302", "49", "L2 Current", "0.009956"], ["150", "4", "303", "50", "L1 Current", "0.009956"], ["151", "4", "304", "50", "L2 Current", "0.008296"], ["152", "4", "305", "51", "L1 Current", "-0.006637"], ["153", "4", "306", "51", "L2 Current", "-0.011615"], ["154", "4", "307", "52", "L1 Current", "0.001659"], ["155", "4", "308", "52", "L2 Current", "0.004978"], ["156", "4", "309", "53", "L1 Current", "0.003319"], ["157", "4", "310", "53", "L2 Current", "0.006637"], ["158", "4", "311", "54", "L1 Current", "0.009956"], ["159", "4", "312", "54", "L2 Current", "0.011615"], ["160", "4", "313", "55", "L1 Current", "0.000000"], ["161", "4", "314", "55", "L2 Current", "0.014933"], ["162", "4", "315", "56", "L1 Current", "0.001659"], ["163", "4", "316", "56", "L2 Current", "0.006637"], ["164", "6", "101", "33", "Temperature", "77.454000"], ["165", "6", "102", "34", "Temperature", "77.456000"], ["166", "6", "103", "35", "Temperature", "77.632000"], ["167", "6", "104", "36", "Temperature", "77.638000"], ["168", "6", "105", "37", "Temperature", "77.159000"], ["169", "6", "106", "38", "Temperature", "75.814000"], ["170", "6", "107", "39", "Temperature", "77.922000"], ["171", "6", "108", "40", "Temperature", "78.196000"], ["172", "6", "109", "41", "Temperature", "78.440000"], ["173", "6", "110", "42", "Temperature", "79.124000"], ["174", "6", "111", "43", "Temperature", "79.366000"], ["175", "6", "112", "44", "Temperature", "79.841000"], ["176", "6", "113", "45", "Temperature", "80.354000"], ["177", "6", "114", "46", "Temperature", "80.293000"], ["178", "6", "115", "47", "Temperature", "80.037000"], ["179", "6", "116", "48", "Temperature", "80.150000"], ["180", "6", "117", "49", "Temperature", "79.992000"], ["181", "6", "118", "50", "Temperature", "80.199000"], ["182", "6", "119", "51", "Temperature", "79.751000"], ["183", "6", "120", "52", "Temperature", "79.949000"], ["184", "6", "201", "53", "Temperature", "80.230000"], ["185", "6", "202", "54", "Temperature", "80.523000"], ["186", "6", "203", "55", "Temperature", "80.593000"], ["187", "6", "204", "56", "Temperature", "1072.373000"], ["188", "6", "205", "33", "Volts", "237.019650"], ["189", "6", "206", "36", "Volts", "236.798560"], ["190", "6", "207", "39", "Volts", "236.814350"], ["191", "6", "208", "42", "Volts", "238.046110"], ["192", "6", "209", "45", "Volts", "230.039650"], ["193", "6", "210", "45", "Volts (208)", "0.536922"], ["194", "6", "211", "45", "SW (208)", "98999999999999993400000000000000000000.000000"], ["195", "6", "212", "48", "Volts", "235.661540"], ["196", "6", "213", "48", "SW (208)", "98999999999999993400000000000000000000.000000"], ["197", "6", "214", "51", "Volts (208)", "199.498200"], ["198", "6", "215", "51", "SW (208)", "98999999999999993400000000000000000000.000000"], ["199", "6", "216", "54", "Volts", "236.135310"], ["200", "6", "301", "17", "Volts", "3.742653"], ["201", "6", "302", "18", "Volts", "0.410586"], ["202", "6", "303", "19", "Volts", "-2.526687"], ["203", "6", "304", "20", "Volts", "-0.900132"], ["204", "6", "305", "51", "Volts", "236.766980"], ["205", "6", "306", "48", "Volts (208)", "199.498200"]]
  in  "file path (dialog if empty)":path=path "C:/Users/220038920/Desktop/Project/NI-2010/Trunk/Dryer Wilt/Documentation/Agilent Array Names.csv"
  in  "Debug":bool
  in  "Index of stations that use\nthe same voltage":string[][](array[string])=[["Station ID (Use Same Voltage Transducer)", "Index in Array", "Agilent Station", "Channel", "Label"], ["21-23", "74", "2", "211", "Volts"], ["24-26", "75", "2", "212", "Volts"], ["27-29", "76", "2", "213", "Volts"], ["30-32", "77", "2", "214", "Volts"], ["33-35", "188", "6", "205", "Volts"], ["36-38", "189", "6", "206", "Volts"], ["39-40", "190", "6", "207", "Volts"], ["42-44", "191", "6", "208", "Volts"], ["45-47", "192", "6", "209", "Volts"], ["48-50", "195", "6", "212", "Volts"], ["54-56", "199", "6", "216", "Volts"], ["51-53", "204", "6", "305", "Volts"]]
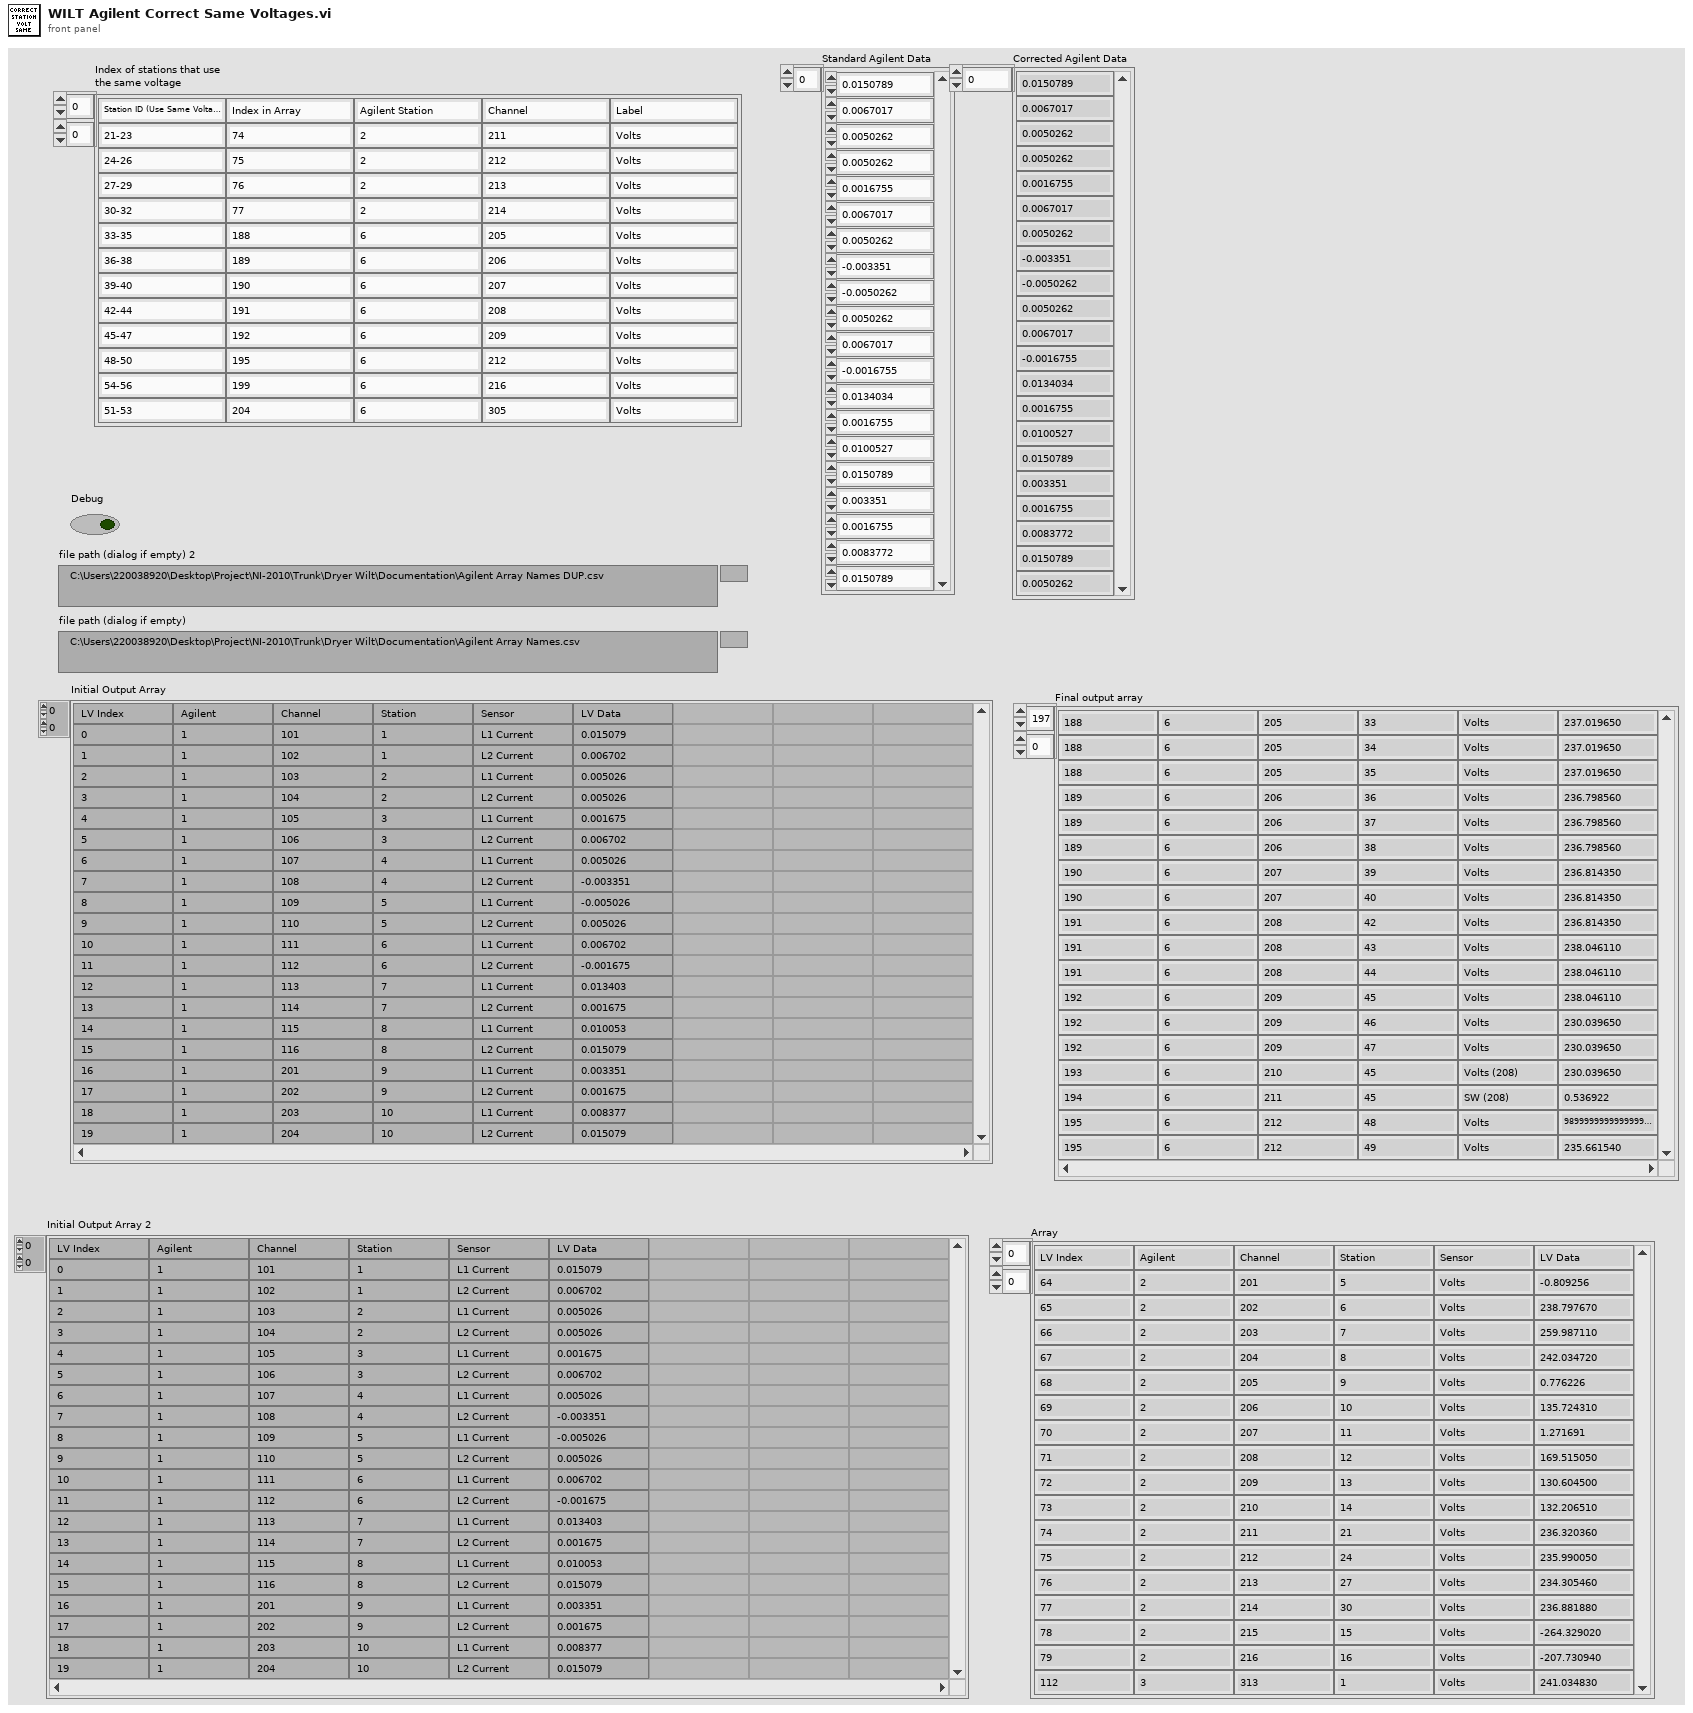
[diagram p1: front panel]
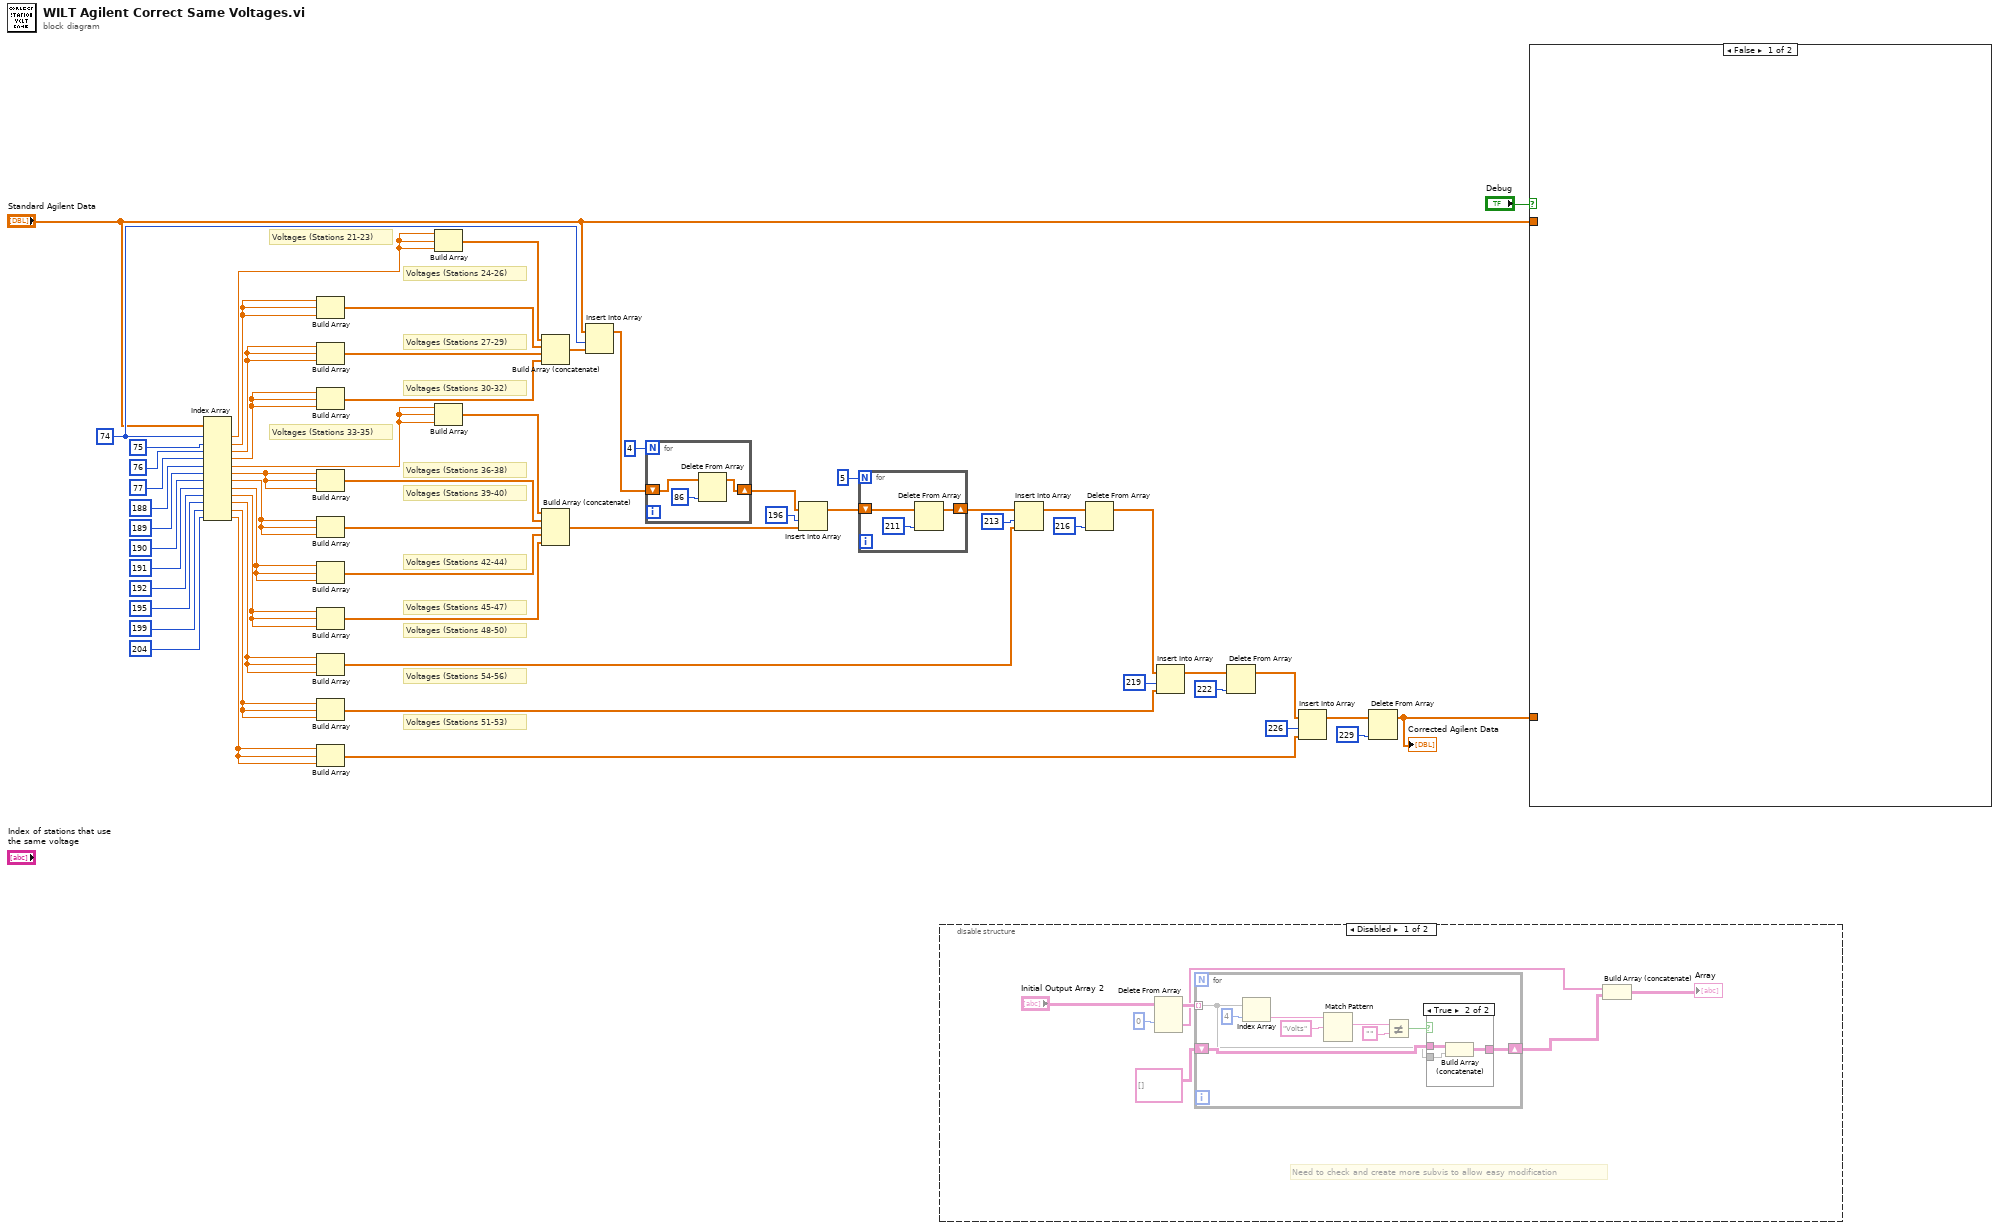
[diagram p0: block diagram]
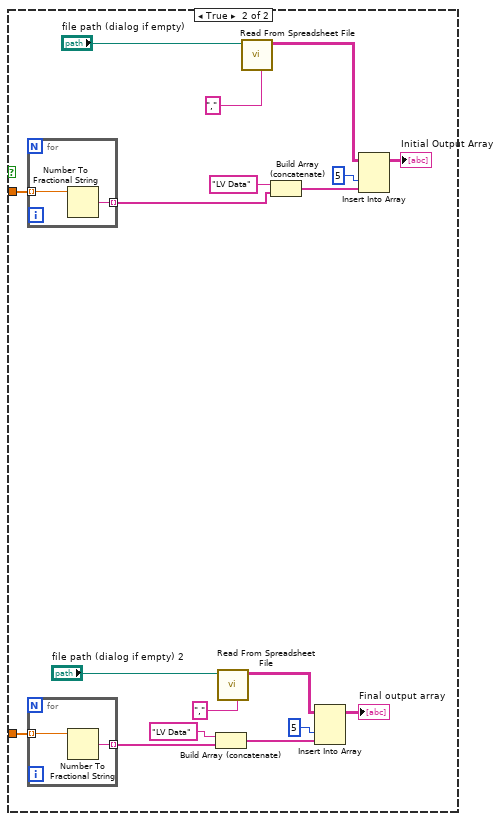
[diagram p4: hidden frame]
diagram:
  w56 = 74 ("index")
  # "Voltages (Stations 51-53)"
  # "Voltages (Stations 54-56)"
  # "Voltages (Stations 48-50)"
  # "Voltages (Stations 45-47)"
  # "Voltages (Stations 42-44)"
  # "Voltages (Stations 39-40)"
  # "Voltages (Stations 36-38)"
  # "Voltages (Stations 33-35)"
  # "Voltages (Stations 30-32)"
  # "Voltages (Stations 27-29)"
  # "Voltages (Stations 24-26)"
  # "Voltages (Stations 21-23)"
  n1 = Index Array(array="Standard Agilent Data", index #1=w56, index #2=75 ("index"), index #3=76 ("index"), index #4=77 ("index"), index #5=188 ("index"), index #6=189 ("index"), index #7=190 ("index"), index #8=191 ("index"), index #9=192 ("index"), index #10=195 ("index"), index #11=199 ("index"), index #12=204 ("index")) -> (element #1=w47:dbl, element #2=w59:dbl, element #3=w58:dbl, element #4=w57:dbl, element #5=w36:dbl, element #6=w35:dbl, element #7=w34:dbl, element #8=w33:dbl, element #9=w32:dbl, element #10=w31:dbl, element #11=w30:dbl, element #12=w29:dbl)
  n2 = Build Array(w59, w59, w59) -> (w51:dbl[])
  n3 = Build Array(w58, w58, w58) -> (w50:dbl[])
  n4 = Build Array(w57, w57, w57) -> (w49:dbl[])
  n5 = Build Array(w35, w35, w35) -> (w27:dbl[])
  n6 = Build Array(w34, w34, w34) -> (w26:dbl[])
  n7 = Build Array(w33, w33, w33) -> (w25:dbl[])
  n8 = Build Array(w32, w32, w32) -> (w24:dbl[])
  n9 = Build Array(w31, w31, w31) -> (w17:dbl[])
  n10 = Build Array(w30, w30, w30) -> (w11:dbl[])
  n11 = Build Array(w29, w29, w29) -> (w6:dbl[])
  n12 = Build Array(w47, w47, w47) -> (w52:dbl[])
  n13 = Build Array(w36, w36, w36) -> (w28:dbl[])
  n14 = Build Array (concatenate)(w52, w51, w50, w49) -> (w48:dbl[])
  n15 = Build Array (concatenate)(w28, w27, w26, w25, w24) -> (w22:dbl[])
  n16 = Insert Into Array(array="Standard Agilent Data", index=w56, new element=w48) -> (w46:dbl[])
  n17 = for {
    N: 4 -> [_]
    shift-right: [w60] -> w21
    shift-left: w46 -> [w61]
    n18 = Delete From Array(array=w61, index=86) -> (array with subset deleted=w60:dbl[])  [unwired: 1 in, 1 out]
  }
  n19 = Insert Into Array(array=w21, index=196, new element=w22) -> (w20:dbl[])
  n20 = for {
    N: 5 -> [_]
    shift-right: [w63] -> w18
    shift-left: w20 -> [w64]
    n21 = Delete From Array(array=w64, index=211) -> (array with subset deleted=w63:dbl[])  [unwired: 1 in, 1 out]
  }
  n22 = disable-structure shown="Disabled" {
    frame Disabled {
      # "Need to check and create more subvis to allow easy modification"
      n23 = Delete From Array(array="Initial Output Array 2", index (row)=0) -> (deleted portion=w67:string[], array with subset deleted=w70:string[][])  [unwired: 2 in]
      n24 = for {
        tunnel: w70 -> [w74] mode=indexing
        shift-right: [w75] -> w68
        shift-left: string[][] [] -> [w76]
        n25 = Index Array(array=w74, index=4) -> (element=w81:string)
        n26 = Match Pattern(string=w81, regular expression="Volts") -> (match substring=w79:string)  [unwired: 1 in, 3 out]
        n27 = Not Equal?(x=w79, y="") -> (x != y?=w77:bool)
        n28 = case shown="True" w77 {
          tunnel: w76 -> [w82 w85]
          tunnel: [w82 w84] -> w75
          tunnel: w74 -> [_ w83]
          frame False {
          }
          frame True {
            n29 = Build Array (concatenate)(w85, w83) -> (w84:string[][])
          }
        }
      }
      n30 = Build Array (concatenate)(w67, w68) -> (→"Array":string[][])
    }
    frame Enabled {
    }
  }
  n31 = Insert Into Array(array=w18, index=213, new element=w17) -> (w15:dbl[])
  n32 = Delete From Array(array=w15, index=216) -> (array with subset deleted=w12:dbl[])  [unwired: 1 in, 1 out]
  n33 = Insert Into Array(array=w12, index=219, new element=w11) -> (w10:dbl[])
  n34 = Delete From Array(array=w10, index=222) -> (array with subset deleted=w7:dbl[])  [unwired: 1 in, 1 out]
  n35 = Insert Into Array(array=w7, index=226, new element=w6) -> (w5:dbl[])
  n36 = Delete From Array(array=w5, index=229) -> (array with subset deleted=w1:dbl[])  [unwired: 1 in, 1 out]
  "Corrected Agilent Data" <- w1
  n37 = case shown="False" "Debug" {
    tunnel: "Standard Agilent Data" -> [_ w103]
    tunnel: w1 -> [_ w94]
    frame False {
    }
    frame True {
      n38 = for {
        tunnel: w103 -> [w107] mode=indexing
        tunnel: [w106] -> w98 mode=indexing
        n39 = Number To Fractional String(number=w107) -> (F-format string=w106:string)  [unwired: 3 in]
      }
      n40 = for {
        tunnel: w94 -> [w105] mode=indexing
        tunnel: [w104] -> w88 mode=indexing
        n41 = Number To Fractional String(number=w105) -> (F-format string=w104:string)  [unwired: 3 in]
      }
      n42 = Build Array (concatenate)("LV Data", w88) -> (w92:string[])
      n43 = call-poly <vilib>:"Read From Spreadsheet File.vi"("delimiter (\\t)"="," ("delimiter (\\t)"), "file path (dialog if empty)"="file path (dialog if empty) 2") -> ("all rows"=w89:string[][])  [unwired: 5 in, 4 out]
      n44 = call-poly <vilib>:"Read From Spreadsheet File.vi"("delimiter (\\t)"="," ("delimiter (\\t)"), "file path (dialog if empty)"="file path (dialog if empty)") -> ("all rows"=w100:string[][])  [unwired: 5 in, 4 out]
      n45 = Build Array (concatenate)("LV Data", w98) -> (w96:string[])
      n46 = Insert Into Array(array=w89, index (col)=5 ("disabled index (col)"), new element=w92) -> (→"Final output array":string[][])  [unwired: 1 in]
      n47 = Insert Into Array(array=w100, index (col)=5 ("disabled index (col)"), new element=w96) -> (→"Initial Output Array":string[][])  [unwired: 1 in]
    }
  }
